vi "AD_Envelope_Generation_subVI.vi"(9 "Release in":i32, 10 "Attack  in":i32, 11 "Number of Samples in":dbl) -> (2 "Envelope XY Graph out":cluster{dbl[], dbl[]}, 3 "Envelope Array out":dbl[](array[numeric]))   [LabVIEW 2024]
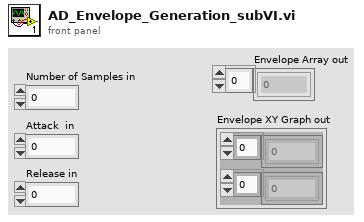
[diagram p1: front panel]
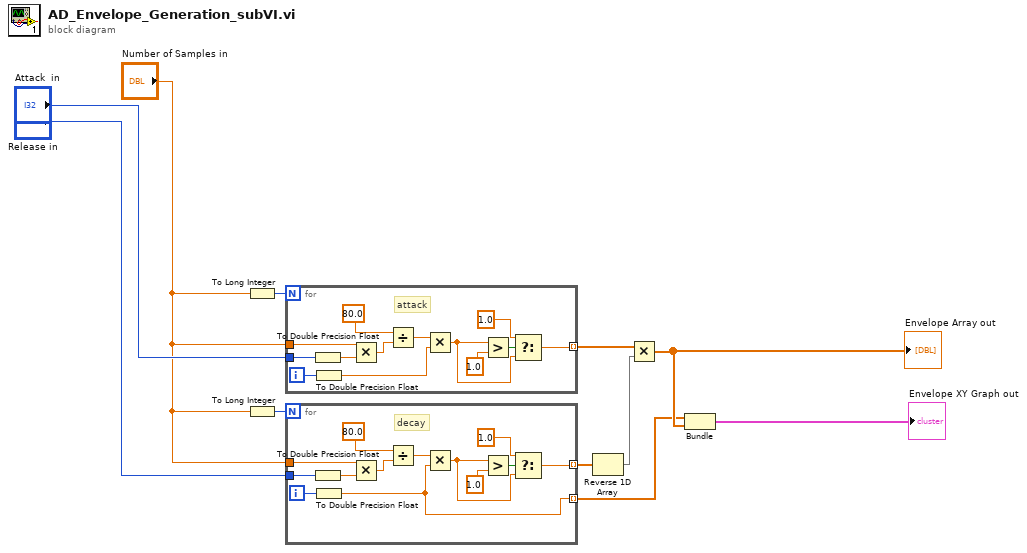
[diagram p0: block diagram]
diagram:
  n1 = To Long Integer(number="Number of Samples in") -> (32bit integer=w1:i32)
  n2 = To Long Integer(number="Number of Samples in") -> (32bit integer=w2:i32)
  n3 = for {
    N: w1 -> [_]
    tunnel: [w15] -> w5 mode=indexing
    tunnel: "Number of Samples in" -> [w14]
    tunnel: "Attack  in" -> [w12]
    i -> [w24]
    # "attack"
    n4 = To Double Precision Float(number=w12) -> (double precision float=w13:dbl)
    n5 = To Double Precision Float(number=w24) -> (double precision float=w17:dbl)
    n6 = Multiply(x=w14, y=w13) -> (x*y=w19:dbl)
    n7 = Divide(x=80.0, y=w19) -> (x/y=w18:dbl)
    n8 = Multiply(x=w18, y=w17) -> (x*y=w16:dbl)
    n9 = Greater?(x=w16, y=1.0) -> (0:w23:bool)
    n10 = Select(t=1.0, s=w23, f=w16) -> (s? t:f=w15:dbl)
  }
  n11 = for {
    N: w2 -> [_]
    tunnel: [w29] -> w4 mode=indexing
    tunnel: "Number of Samples in" -> [w28]
    tunnel: [w26] -> w7 mode=indexing
    tunnel: "Release in" -> [w25]
    i -> [w37]
    # "decay"
    n12 = To Double Precision Float(number=w25) -> (double precision float=w27:dbl)
    n13 = To Double Precision Float(number=w37) -> (double precision float=w26:dbl)
    n14 = Multiply(x=w28, y=w27) -> (x*y=w32:dbl)
    n15 = Divide(x=80.0, y=w32) -> (x/y=w31:dbl)
    n16 = Multiply(x=w31, y=w26) -> (x*y=w30:dbl)
    n17 = Greater?(x=w30, y=1.0) -> (0:w36:bool)
    n18 = Select(t=1.0, s=w36, f=w30) -> (s? t:f=w29:dbl)
  }
  n19 = Reverse 1D Array(array=w4) -> (reversed array=w6:dbl[])
  n20 = Multiply(x=w5, y=w6) -> (x*y=w11:dbl[])
  "Envelope Array out" <- w11
  n21 = Bundle(w7, w11) -> (→"Envelope XY Graph out":cluster{dbl[], dbl[]})  [unwired: 1 in]
